vi "AsyncEngine.GhostBus.vi"(10 "Parameters":variant, 11 "Process":refnum<class "Process.lvclass">) -> ()   [LabVIEW 2019, in "Ghost Bus Addon Engine.lvlib"]
uses:
  Ghost Bus Addon Engine.lvlib
  <vilib>/Platform/TimedLoop/XDataNode/XDataNode.xnode
  <vilib>/Platform/TimedLoop/XDataNode/timing_clust.ctl
  <vilib>/Platform/TimedLoop/XDataNode/XDNodeRunTimeDep.lvlib
  <vilib>/Platform/TimedLoop/XDataNode/wakeup.ctl
  <vilib>/Platform/TimedLoop/XDataNode/nitl_modes.ctl
  <vilib>/NI/NIVS Inline Async API/_VS Inline Async API/Process/Process.lvclass
  SubModules/CAN-Streaming-Support/Source/Addon/Addon Engine/CAN Stream Support Engine.lvlib
  Types/RT XNET Refs.ctl
  Types/RT Bus Settings.ctl
  Addon Shared/Types/XNET Port Settings.ctl
  Addon Shared/Ghost Bus Addon Shared.lvlib
  <vilib>/NI/NIVS Inline Async API/_Data Access Engine/Data Access Engine/Data Access Engine.lvclass
  <vilib>/NI/NIVS Inline Async API/_Data Access Engine/Data Access Engine/Methods/Write.Data.vi
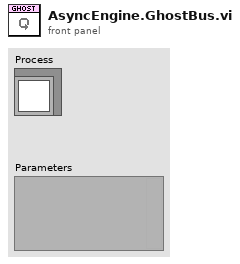
[diagram p1: front panel]
types:
  T1 = typedef "RT Bus Settings.ctl" = cluster{"Name":string, "Overrides?":bool, "XNET Refs":T2, "Port Info":T3, "Frames":variant}
  T2 = typedef "Ghost Bus Addon Engine.lvlib/RT XNET Refs.ctl" = cluster{"Incoming":refnum<k21>, "Outgoing":refnum<k21>}
  T3 = typedef "Ghost Bus Addon Shared.lvlib/XNET Port Settings.ctl" = cluster{"Port":string, "Baud Rate":u64, "Termination":u32, "CAN I/O Mode":u32, "FD Baud Rate":u64, "Priority":i32, "FD ISO Mode":u32}
  T4 = typedef "Ghost Bus Addon Engine.lvlib/RT Async Engine Variables.ctl" = cluster{"Process Ref":refnum<class "Process.lvclass">, "Comm Ref":refnum<class "VeriStand Comm.lvclass">, "Bus Info":T1, "Stream Refs":T5, "Data Refs":T10}
  T5 = typedef "CAN Stream Support Engine.lvlib/Engine Stream Refs.ctl" = cluster{"Addon":string, "Port":refnum<k21>, "Filter Ref":refnum<data-value>, "Default Filter":T6, "Port Settings":T9}
  T6 = typedef "CAN Stream Support Shared.lvlib/Filter Parameters.ctl" = cluster{"ID Filters":u32[], "Direction Filter":T7, "Type Filter":T8}
  T7 = typedef "CAN Stream Support Shared.lvlib/Direction Filter.ctl" = enum16{"Tx/Rx", "Rx", "Tx"}
  T8 = typedef "CAN Stream Support Shared.lvlib/Type Filter.ctl" = enum16{"All", "CAN Data", "CAN Remote", "CAN Bus Error", "CAN 2.0 Data", "CAN FD Data", "CAN FD+BRS Data", "J1939 Data", "Delay", "Log Trigger", "Start Trigger"}
  T9 = typedef "CAN Stream Support Engine.lvlib/Engine Stream Port Settings.ctl" = cluster{"Mode":u32, "Baud Rate":u64, "Termination":u32, "FD ISO Mode":u32, "FD Baud Rate":u64}
  T10 = typedef "Ghost Bus Addon Engine.lvlib/RT Data Refs.ctl" = cluster{"Port.Status":T11, "Frame.Enable":T12, "Frame.Signals":T12, "Frame.Overrides":T12, "Port.Enable":T12}
  T11 = typedef "Data Access Engine.lvlib/Data Access Engine.lvclass/Write.DVR.ctl" = refnum<data-value>
  T12 = typedef "Data Access Engine.lvlib/Data Access Engine.lvclass/Read.DVR.ctl" = refnum<data-value>
  T13 = typedef "XDNodeRunTimeDep.lvlib/timing_clust.ctl" = cluster{"Expected End [f-1]":u64, "Actual End [f-1]":u64, "Finished Late? [f-1]":bool, "Expected End [i-1]":u64, "Actual End [i-1]":u64, "Finished Late? [i-1]":bool, "Expected Start [i]":u64, "Actual Start [i]":u64, "Expected Start [f]":u64, "Actual Start [f]":u64, "Source Name":string, "Structure Name":string, "Period":i64, "Deadline":i64, "Offset":i64, "Start":i64, "Priority":i32, "Timeout":i32, "Mode":T14, "Wakeup Reason":T15, "Error":errorcluster, "Source Type":string, "Secondary Source Type":string, "Global End Time":u64, "Global Start Time":u64, "Frame Duration":u64, "Iteration Duration":u64, "Assigned CPU":i32, "I/O Scan Engine Mode":u32}
  T14 = typedef "XDNodeRunTimeDep.lvlib/nitl_modes.ctl" = enum32{"No Change", "Process missed periods, maintain original phase", "Discard missed periods, maintain original phase", "Process missed periods, ignore original phase", "Discard missed periods, ignore original phase"}
  T15 = typedef "XDNodeRunTimeDep.lvlib/wakeup.ctl" = enum32{"Normal", "Aborted", "Asynchronous wakeup", "Timing source error", "Timed loop error", "Timeout"}
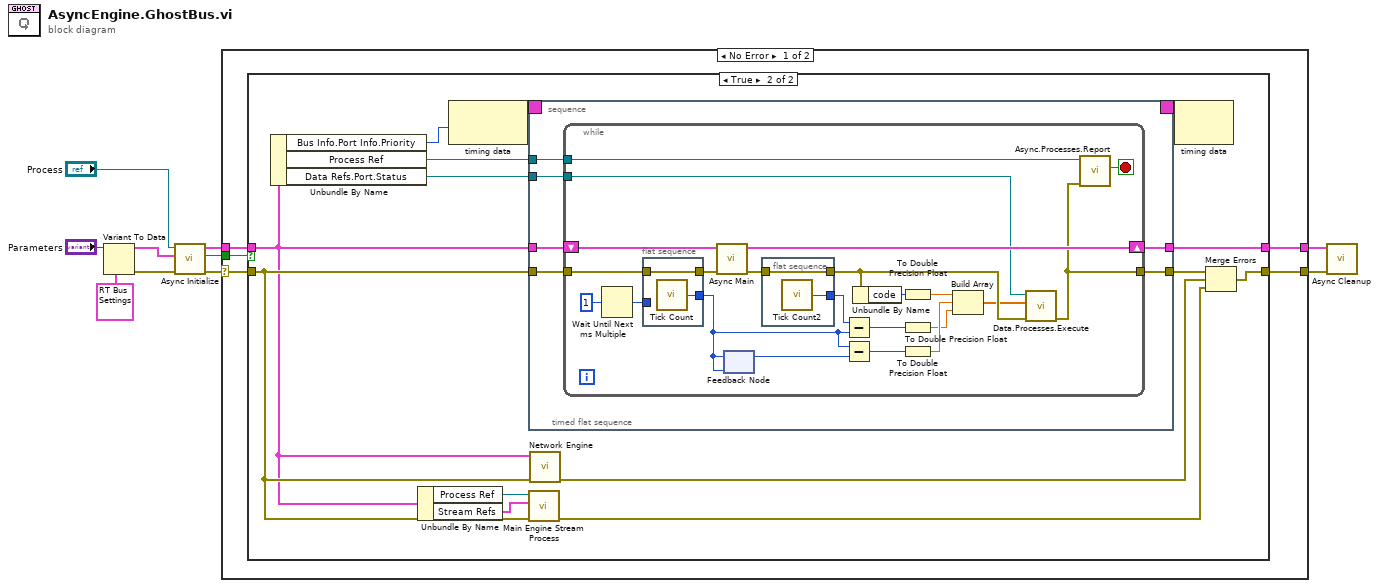
[diagram p0: block diagram]
diagram:
  n1 = Variant To Data(type=T1 {"Name"="", "Overrides?"=FALSE, "XNET Refs"={"Incoming"="", "Outgoing"=""}, "Port Info"={"Port"="", "Baud Rate"=0, "Termination"=0, "CAN I/O Mode"=0, "FD Baud Rate"=500000, "Priority"=100, "FD ISO Mode"=0}, "Frames"=variant(cluster{"Convert Session":refnum<k21>, "ID":u32, "Length":i32, "Offset":i32}[] [])} ("Bus Settings"), Variant="Parameters") -> (data=w2:T1, error out=w6:errorcluster)  [unwired: 1 in]
  n2 = call "Async Initialize.vi"("error in (no error)"=w6, "Bus Settings"=w2, "Process in"="Process") -> ("error out"=w3:errorcluster, "Execute"=w5:bool, "Variables"=w4:T4)  [unwired: 6 in]
  n3 = case shown="No Error" w3 {
    selector: w3 -> [w14 w77]
    tunnel: w5 -> [w15 _]
    tunnel: [w13 w77] -> w7
    tunnel: [w12 w76] -> w8
    tunnel: w4 -> [w11 w76]
    frame No Error {
      n4 = case shown="True" w15 {
        tunnel: w14 -> [w17 w22]
        tunnel: [w17 w26] -> w13
        tunnel: [w16 w31] -> w12
        tunnel: w11 -> [w16 w20]
        frame False {
        }
        frame True {
          n5 = Unbundle By Name(w20) -> ("Bus Info.Port Info.Priority"=w28:i32, "Process Ref"=w27:refnum<class "Process.lvclass">, "Data Refs.Port.Status"=w18:T11)
          n6 = Unbundle By Name(w20) -> ("Process Ref"=w24:refnum<class "Process.lvclass">, "Stream Refs"=w23:T5)
          n7 = node-c288(w28) -> (w30:T13)
          n8 = timed-sequence {
            timing: w30 -> [_]
            timing-out: [_] -> w29
            tunnel: w27 -> [w33]
            tunnel: w20 -> [w35]
            tunnel: w22 -> [w34]
            tunnel: [w37] -> w19
            tunnel: [w36] -> w31
            tunnel: w18 -> [w32]
            n9 = timed-flat-sequence {
              tunnel: [w39] -> w37
              tunnel: [w40] -> w36
              tunnel: w35 -> [w43]
              tunnel: w34 -> [w42]
              tunnel: w33 -> [w41]
              tunnel: w32 -> [w38]
              n10 = while {
                tunnel: w41 -> [w65]
                tunnel: w42 -> [w59]
                shift-right: [w63] -> w40
                shift-left: w43 -> [w62]
                tunnel: [w47] -> w39
                tunnel: w38 -> [w61]
                stop <- w64 stop-if-true
                n11 = Wait Until Next ms Multiple(millisecond multiple=u32 1) -> (millisecond timer value=w45:u32)
                n12 = flat-sequence {
                  tunnel: [w69] -> w56
                  tunnel: [w68] -> w58
                  tunnel: w59 -> [w68]
                  tunnel: w45 -> [_]
                  frame #0 {
                    n13 = call "Tick Count"() -> ("Tick Count(uSec)"=w69:u32)
                  }
                }
                n14 = call "Async Main.vi"("error in (no error)"=w58, "Variables in"=w62) -> ("error out"=w60:errorcluster, "Variables out"=w63:T4)  [unwired: 8 in]
                n15 = feedback #1(w56) -> (w55:u32)
                n16 = feedback-in #1(w56) -> ()
                n17 = flat-sequence {
                  tunnel: [w67] -> w57
                  tunnel: w60 -> [w66]
                  tunnel: [w66] -> w48
                  frame #0 {
                    n18 = call "Tick Count2"() -> ("Tick Count(uSec)"=w67:u32)
                  }
                }
                n19 = Subtract(x=w57, y=w56) -> (x-y=w53:u32)
                n20 = Subtract(x=w56, y=w55) -> (x-y=w52:u32)
                n21 = Unbundle By Name(w48) -> ("code"=w54:i32)
                n22 = To Double Precision Float(number=w54) -> (double precision float=w51:dbl)
                n23 = To Double Precision Float(number=w53) -> (double precision float=w49:dbl)
                n24 = To Double Precision Float(number=w52) -> (double precision float=w50:dbl)
                n25 = Build Array(w51, w50, w49) -> (w46:dbl[])
                n26 = call-poly <vilib>:"Data.Processes.Execute.vi"("error in (no error)"=w48, "Values"=w46, "Ref"=w61) -> ("error out"=w47:errorcluster)  [unwired: 8 in]
                n27 = call <vilib>:"Async.Processes.Report.vi"("Error"=w47, "Process in"=w65) -> ("Stop"=w64:bool)  [unwired: 8 in, 1 out]
              }
            }
          }
          n28 = call "Main Engine Stream Process.vi"("error in (no error)"=w22, "Refs"=w23, "Process in"=w24) -> ("error out"=w21:errorcluster)  [unwired: 8 in]
          n29 = call "Network Engine.vi"("error in (no error)"=w22, "Variables"=w20) -> ("error out"=w25:errorcluster)  [unwired: 9 in]
          n30 = node-c288(w29) -> ()  [unwired: 1 out]
          n31 = Merge Errors(w19, w25, w21) -> (w26:errorcluster)
        }
      }
    }
    frame Error {
    }
  }
  n32 = call "Async Cleanup.vi"("error in (no error)"=w7, "Variables"=w8) -> ()  [unwired: 9 in, 1 out]
